vi "Format ProductCodesSetItemType_LVXML_Loop.vi"(8 "error in (no error)":errorcluster, 10 "Siblings in 3":T3(array[cluster]), 11 "AWS_EC2 in":refnum<class "AWS_EC2.lvclass">) -> (0 "error out":errorcluster, 2 "Array":T1[](array[typedef]), 3 "AWS_EC2 out":refnum<class "AWS_EC2.lvclass">)   [LabVIEW 2014, in "AWS_EC2.lvlib" / "AWS_EC2.lvclass"]
uses:
  AWS_EC2.lvclass
  lv-xml-parser/r0/trunk/VI Source/EventType.ctl
  EC2 Datatypes/ProductCodeSetItemType.ctl
  AWS_EC2.lvlib
  lv-xml-parser/r0/trunk/VI Source/LV XML Parser.lvlib
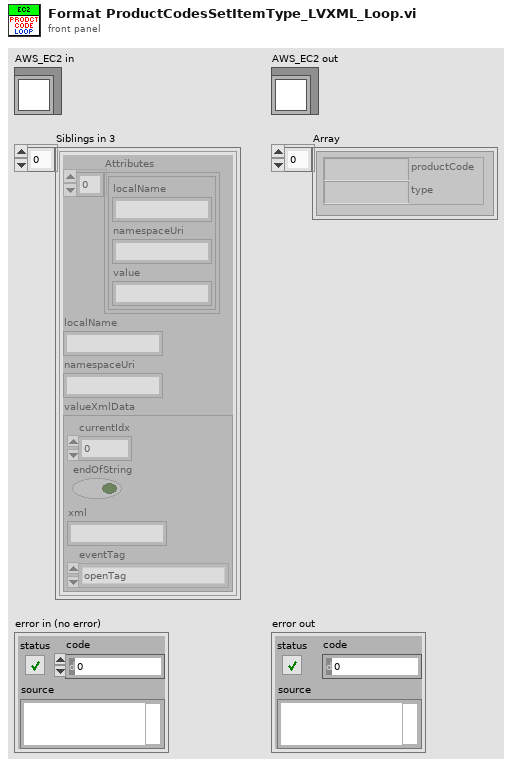
[diagram p1: front panel]
types:
  T1 = typedef "AWS_EC2.lvlib/ProductCodeSetItemType.ctl" = cluster{"productCode":string, "type":string}
  T2 = typedef "LV XML Parser.lvlib/EventType.ctl" = enum16{"openTag", "endOpenTag", "closeTag", "comment", "endComment", "endOfFile", "attribute", "startXml"}
  T3 = cluster{"Attributes":cluster{"localName":string, "namespaceUri":string, "value":string}[], "localName":string, "namespaceUri":string, "valueXmlData":cluster{"currentIdx":i32, "endOfString":bool, "xml":string, "eventTag":T2}}[]
  T4 = cluster{"Attributes":cluster{"localName":string, "namespaceUri":string, "value":string}[], "localName":string, "namespaceUri":string, "valueXmlData":cluster{"currentIdx":i32, "endOfString":bool, "xml":string, "eventTag":T2}}
  T5 = cluster{"currentIdx":i32, "endOfString":bool, "xml":string, "eventTag":T2}
  T6 = cluster{"namespaceUri":string, "localName":string}
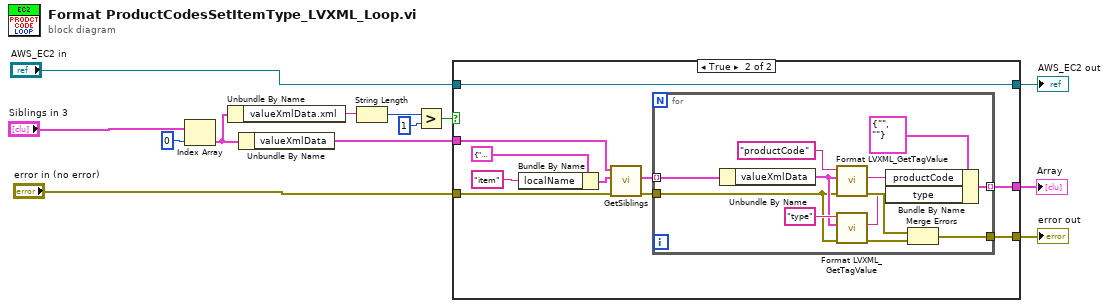
[diagram p0: block diagram]
diagram:
  n1 = Index Array(array="Siblings in 3", index=0) -> (element=w4:T4)
  n2 = Unbundle By Name(w4) -> ("valueXmlData.xml"=w5:string)
  n3 = Unbundle By Name(w4) -> ("valueXmlData"=w6:T5)
  n4 = String Length(string=w5) -> (length=w9:i32)
  n5 = Greater?(x=w9, y=1) -> (0:w7:bool)
  n6 = case shown="True" w7 {
    tunnel: [w15 w24] -> w13
    tunnel: "error in (no error)" -> [w15 w19]
    tunnel: w6 -> [_ w18]
    tunnel: "AWS_EC2 in" -> [w14 w17]
    tunnel: [w14 w17] -> w2
    tunnel: [_ w16] -> w1
    frame False {
    }
    frame True {
      n7 = Bundle By Name(cluster=T6 {"namespaceUri"="", "localName"=""} ("limitToTag"), "localName"="item" ("Tag name")) -> (w21:T6)
      n8 = call "GetSiblings.vi"("error in (no error)"=w19, "limitToTag"=w21, "xmlData"=w18) -> ("error out"=w25:errorcluster, "Siblings"=w22:T3)  [unwired: 7 in]
      n9 = for {
        tunnel: w22 -> [w37] mode=indexing
        tunnel: [w36] -> w24
        tunnel: w25 -> [w30]
        tunnel: [w29] -> w16 mode=indexing
        n10 = Unbundle By Name(w37) -> ("valueXmlData"=w33:T5)
        n11 = call "Format LVXML_GetTagValue.vi"("error in (no error)"=w30, "xmlDataIn"=w33, "Tag name"="productCode") -> ("error out"=w32:errorcluster, "Value"=w27:string)  [unwired: 6 in, 1 out]
        n12 = call "Format LVXML_GetTagValue.vi"("error in (no error)"=w30, "xmlDataIn"=w33, "Tag name"="type") -> ("error out"=w31:errorcluster, "Value"=w28:string)  [unwired: 6 in, 1 out]
        n13 = Bundle By Name(cluster=T1 {"productCode"="", "type"=""} ("ProductCodesSetItemType"), "productCode"=w27, "type"=w28) -> (w29:T1)
        n14 = Merge Errors(w32, w31) -> (w36:errorcluster)
      }
    }
  }
  "error out" <- w13
  "AWS_EC2 out" <- w2
  "Array" <- w1
